vi "Report Generation.vi"() -> ()   [LabVIEW 2021, in "User Interface.lvlib"]
uses:
  User Interface.lvlib
  <vilib>/Utility/miscctls.llb/LVPointTypeDef.ctl
  Testing Command.ctl
  Report Datahighway.ctl
  VI Name.ctl
  Database/Database.lvlib
panel:
  in  "Search":bool
  in  "To":timestamp
  in  "From":timestamp
  out "Table Control":string[][](table)
  in  "EXIT":bool
  out "error out":errorcluster
  in  "error in (no error)":errorcluster
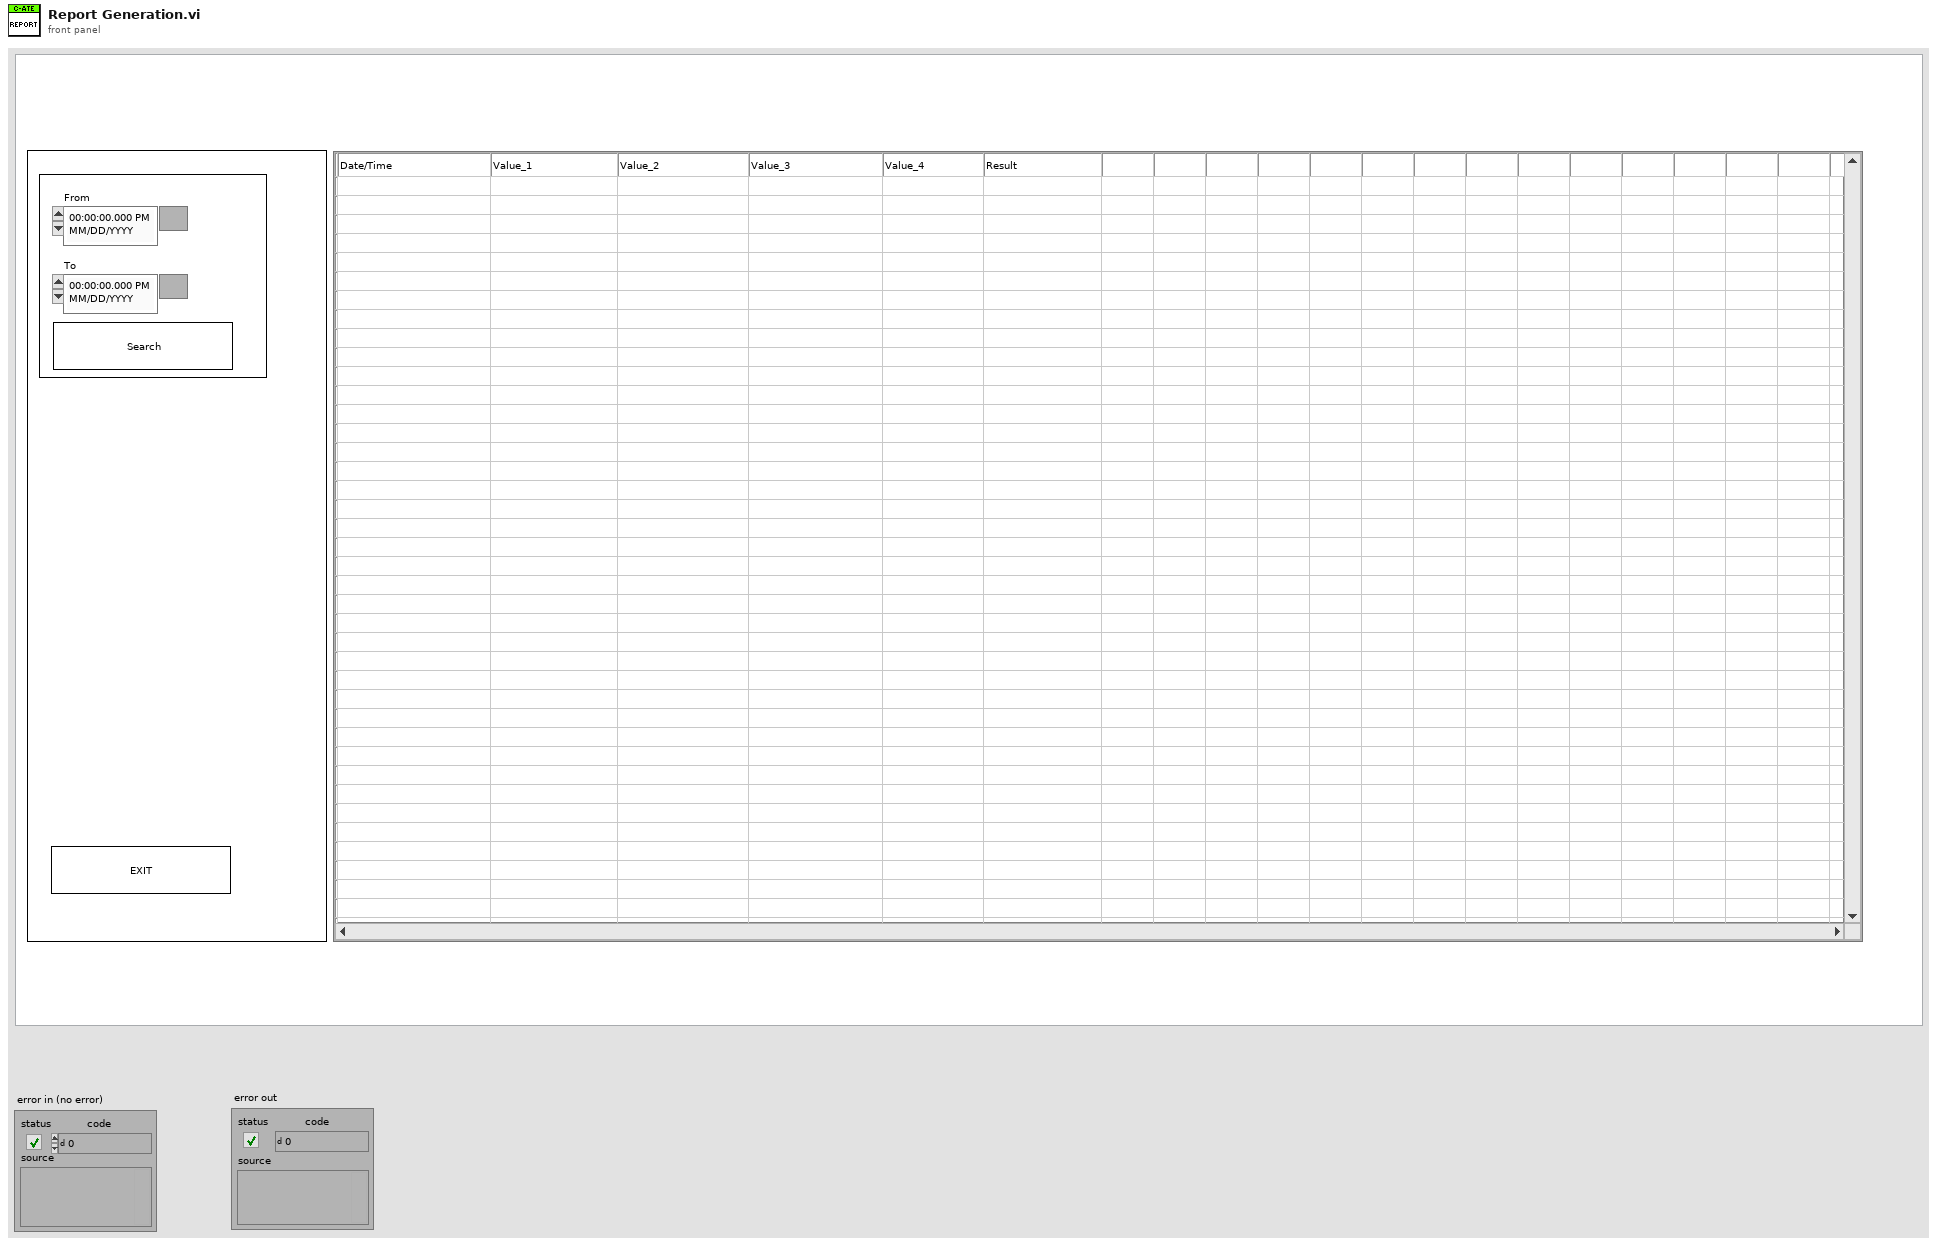
[diagram p1: front panel]
types:
  T1 = typedef "User Interface.lvlib/Report Datahighway.ctl" = cluster{"Report Data":string[][]}
  T2 = typedef "User Interface.lvlib/Testing Command.ctl" = enum16{"Init", "Main", "Close"}
  T3 = typedef "LVPointTypeDef.ctl" = cluster{"Horizontal":i16, "Vertical":i16}
  T4 = typedef "User Interface.lvlib/VI Name.ctl" = enum16{"Dashboard", "Maintenance", "Recipe", "Inst Configuration", "Testing", "Report"}
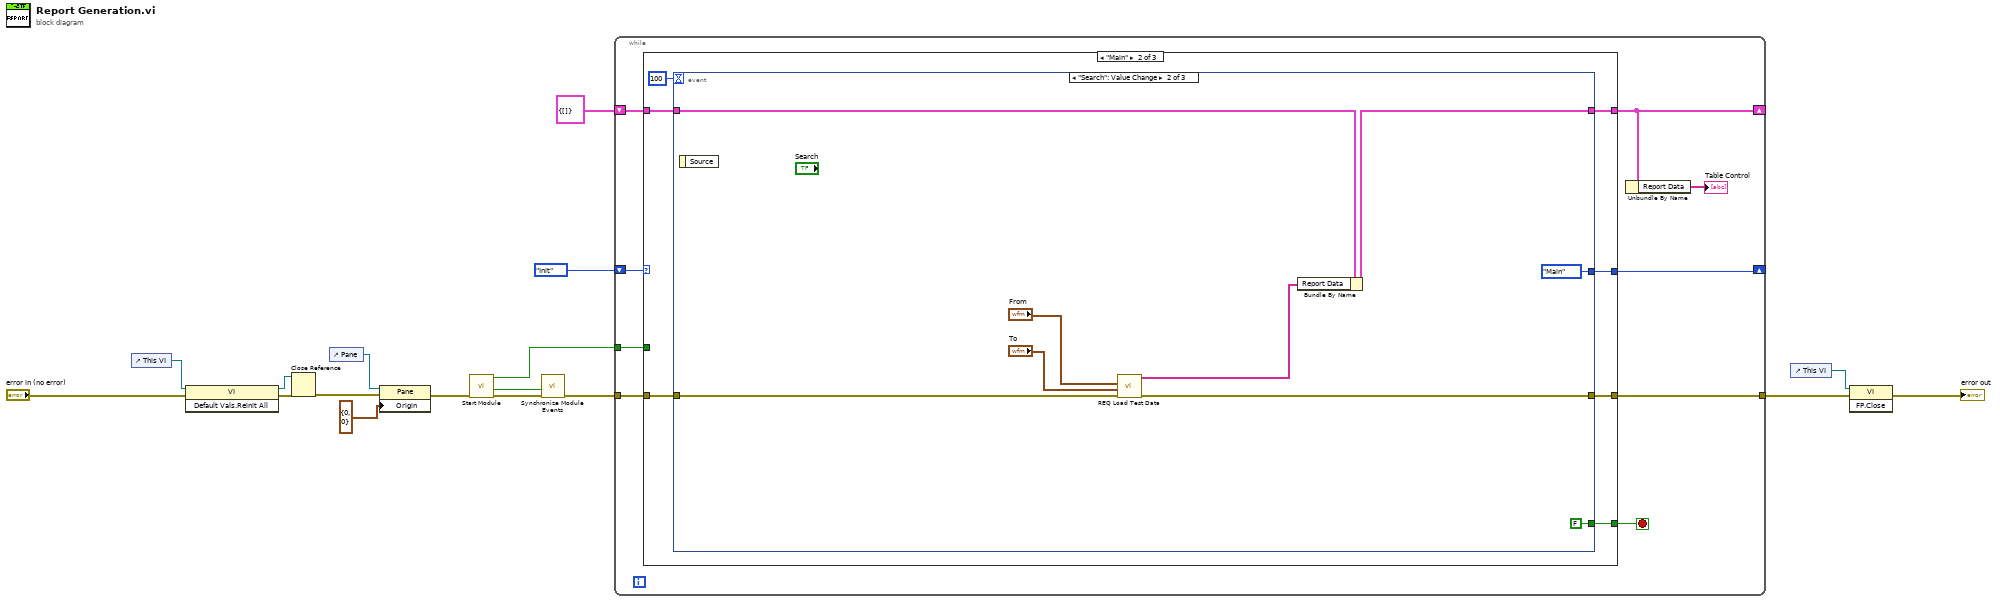
[diagram p0: block diagram]
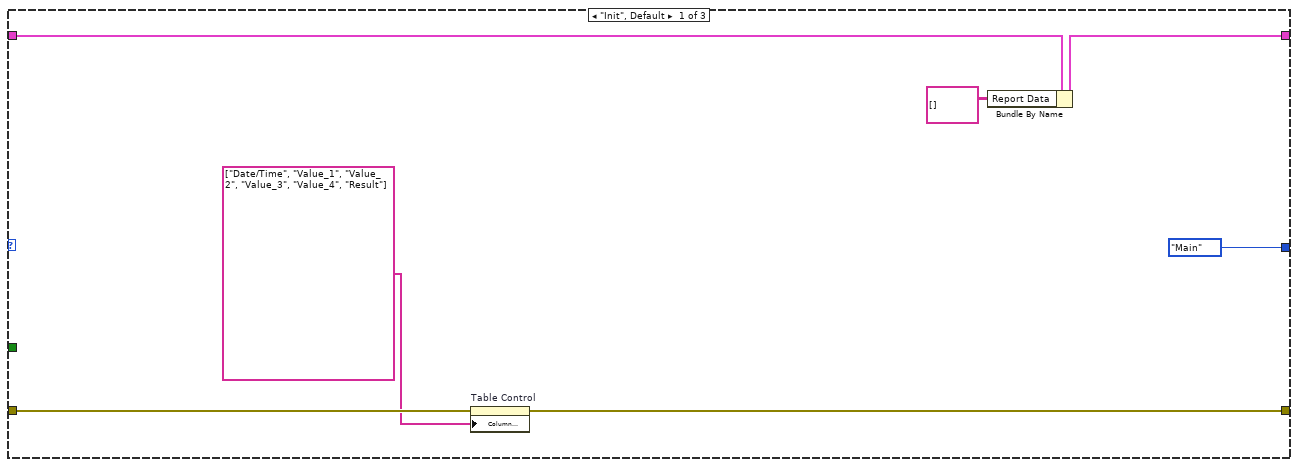
[diagram p2: hidden frame]
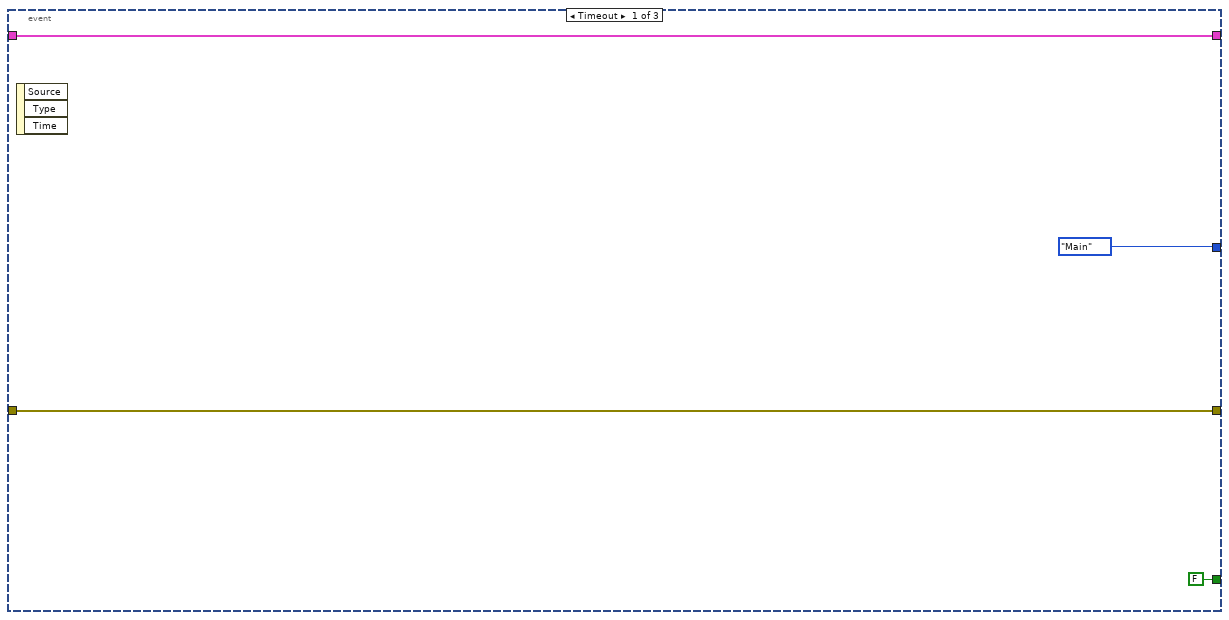
[diagram p3: hidden frame]
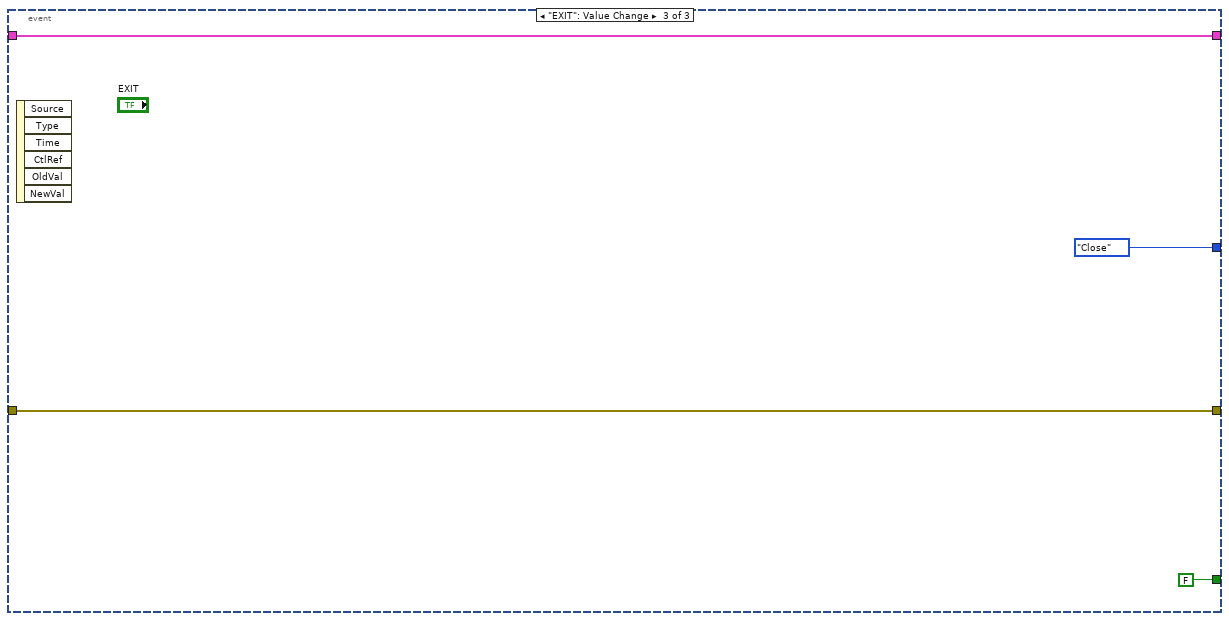
[diagram p4: hidden frame]
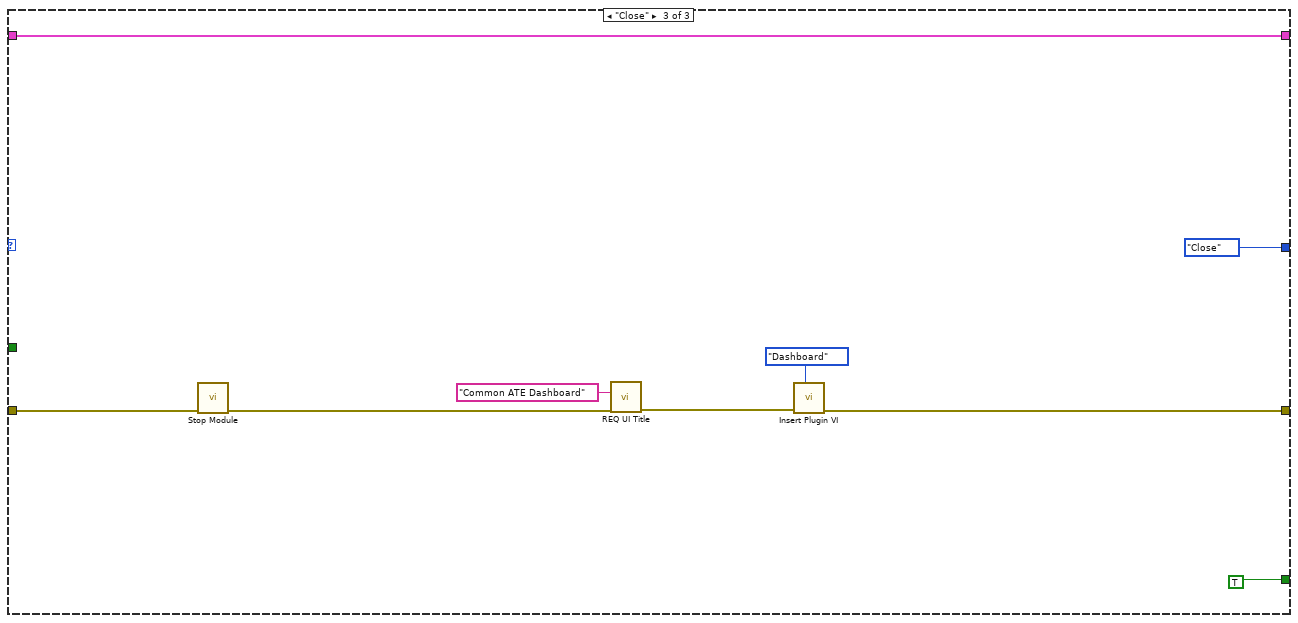
[diagram p5: hidden frame]
diagram:
  n1 = control-ref of="This VI"() -> (w13:refnum<vi>)
  n2 = invoke class="VI" method="Default Vals.Reinit All"(reference=w13, error in="error in (no error)") -> (reference out=w11:refnum<vi>, error out=w12:errorcluster)  [unwired: 1 in, 1 out]
  n3 = Close Reference(reference=w11, error in (no error)=w12) -> (error out=w9:errorcluster)
  n4 = control-ref of="Pane"() -> (w7:refnum<vi>)
  n5 = property class="Pane"(reference=w7, error in=w9, "Origin"=T3 {"Horizontal"=0, "Vertical"=0}) -> (error out=w4:errorcluster)  [unwired: 1 out]
  n6 = call "Start Module.vi"("error in"=w4) -> ("error out"=w6:errorcluster, "Wait for Event Sync?"=w5:bool, "Module Was Already Running?"=w2:bool)  [unwired: 7 in, 1 out]
  n7 = call "Synchronize Module Events.vi"("error in"=w6, "Wait for Event Sync?"=w5) -> ("error out"=w3:errorcluster)  [unwired: 9 in]
  n8 = while {
    tunnel: w3 -> [w26]
    shift-right: [w22] -> _
    shift-left: Testing_Command."Init" -> [w25]
    tunnel: [w24] -> w15
    tunnel: w2 -> [w21]
    shift-right: [w19] -> _
    shift-left: T1 {"Report Data"=[]} -> [w20]
    stop <- w23 stop-if-true
    n9 = case shown="\"Main\"" w25 {
      tunnel: w26 -> [w32 w39 w60]
      tunnel: [w31 w38 w65] -> w24
      tunnel: [_ w37 TRUE] -> w23
      tunnel: [Testing_Command."Main" w36 Testing_Command."Close"] -> w22
      tunnel: w21 -> [_ _ _]
      tunnel: w20 -> [w29 w35 w58]
      tunnel: [w28 w34 w58] -> w19
      frame "Init", Default {
        n10 = property on="Table Control" class="Tbl (strict)"(error in=w32, "Column Headers[]"=string[] ["Date/Time", "Value_1", "Value_2", "Value_3", "Value_4", "Result"]) -> (error out=w31:errorcluster)  [unwired: 1 in, 1 out]
        n11 = Bundle By Name(cluster=w29, "Report Data"=string[][] []) -> (w28:T1)
      }
      frame "Main" {
        n12 = event shown="[1] \"Search\": Value Change" {
          selector: _ -> [_ _ _]
          dyn-events: _ -> [_ _ _]
          timeout: 100 -> [_ _ _]
          tunnel: w39 -> [w44 w53 w57]
          tunnel: [w44 w51 w57] -> w38
          tunnel: [FALSE FALSE FALSE] -> w37
          tunnel: [Testing_Command."Main" ("Command") Testing_Command."Main" Testing_Command."Close"] -> w36
          tunnel: w35 -> [w42 w52 w54]
          tunnel: [w42 w47 w54] -> w34
          event Timeout {
            n13 = event-data() -> ()  [unwired: 1 in, 3 out]
          }
          event "Search": Value Change {
            n14 = event-data() -> ()  [unwired: 1 in, 1 out]
            n15 = call "REQ Load Test Data.vi"("error in"=w53, "To"="To", "From"="From") -> ("error out"=w51:errorcluster, "Test Data"=w46:string[][])  [unwired: 6 in, 1 out]
            n16 = Bundle By Name(cluster=w52, "Report Data"=w46) -> (w47:T1)
          }
          event "EXIT": Value Change {
            n17 = event-data() -> ()  [unwired: 1 in, 6 out]
          }
        }
      }
      frame "Close" {
        n18 = call "Stop Module.vi"("error in"=w60) -> ("error out"=w59:errorcluster)  [unwired: 10 in]
        n19 = call "REQ UI Title.vi"("error in"=w59, "UI Title"="Common ATE Dashboard" ("ATE Title")) -> ("error out"=w61:errorcluster)  [unwired: 9 in]
        n20 = call "Insert Plugin VI.vi"("VI Name"=VI_Name."Dashboard", "error in (no error)"=w61) -> ("error out"=w65:errorcluster)  [unwired: 9 in]
      }
    }
    n21 = Unbundle By Name(w19) -> ("Report Data"=→"Table Control":string[][])
  }
  n22 = control-ref of="This VI"() -> (w16:refnum<vi>)
  n23 = invoke class="VI" method="FP.Close"(reference=w16, error in=w15) -> (error out=→"error out":errorcluster)  [unwired: 1 in, 2 out]
